vi "StopAcquisition.vi"(8 "error in (no error)":errorcluster, 11 "reference in":refnum<class "Camera_IMAQdx.lvclass">) -> (0 "error out":errorcluster, 3 "reference out":refnum<class "Camera_IMAQdx.lvclass">)   [LabVIEW 2017, in "Camera_IMAQdx.lvclass"]
doc: "Starts IMAQdx Acquisition. Use this with Grab when you are done getting images."
uses:
  Camera_IMAQdx.lvclass
  <vilib>/vision/driver/NI_Vision_Acquisition_Software.lvlib
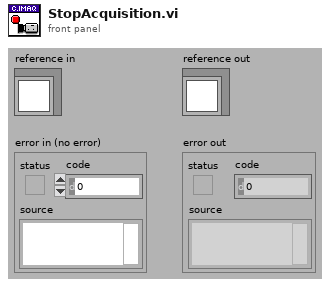
[diagram p1: front panel]
types:
  T1 = typedef "IMAQdx.ctl" = refnum<k21>
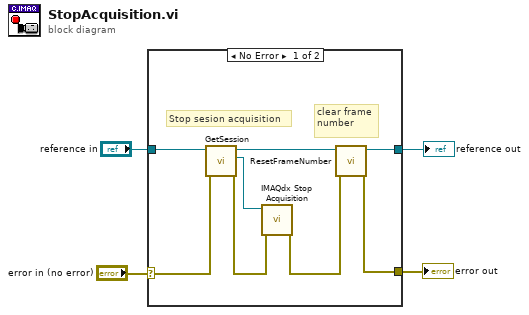
[diagram p0: block diagram]
diagram:
  n1 = case shown="No Error" "error in (no error)" {
    selector: "error in (no error)" -> [w10 w14]
    tunnel: [w5 w14] -> w3
    tunnel: [w7 w13] -> w1
    tunnel: "reference in" -> [w12 w13]
    frame No Error {
      # "clear frame number"
      # "Stop sesion acquisition"
      n2 = call "GetSession.vi"("error in (no error)"=w10, "reference in"=w12) -> ("error out"=w9:errorcluster, "Session"=w11:T1, "reference out"=w8:refnum<class "Camera_IMAQdx.lvclass">)  [unwired: 7 in]
      n3 = call <vilib>:"IMAQdx Stop Acquisition.vi"("error in"=w9, "Session In"=w11) -> ("error out"=w6:errorcluster)  [unwired: 8 in, 1 out]
      n4 = call "ResetFrameNumber.vi"("error in (no error)"=w6, "reference in"=w8) -> ("error out"=w5:errorcluster, "reference out"=w7:refnum<class "Camera_IMAQdx.lvclass">)  [unwired: 8 in]
    }
    frame Error {
    }
  }
  "error out" <- w3
  "reference out" <- w1
